vi "To XML - Returns XML Entities.vi"() -> ()   [LabVIEW 2017, in "Cobertura.Tests.lvlib" / "Class.lvlib"]
uses:
  Class.lvlib
  <vilib>/xml/Close Reference(Node).vi
  Cobertura/Class/Class.lvclass
  <vilib>/xml/NI_XML.lvlib
  <resource>/objmgr/DOMUserDefRef.rc
  <vilib>/PNR/Transparent Assertions/Transparent Assertions/Transparent Assertions.lvlib
panel:
  out "error out":errorcluster
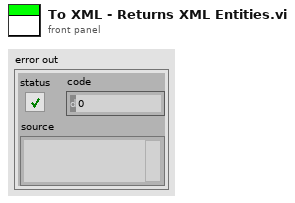
[diagram p1: front panel]
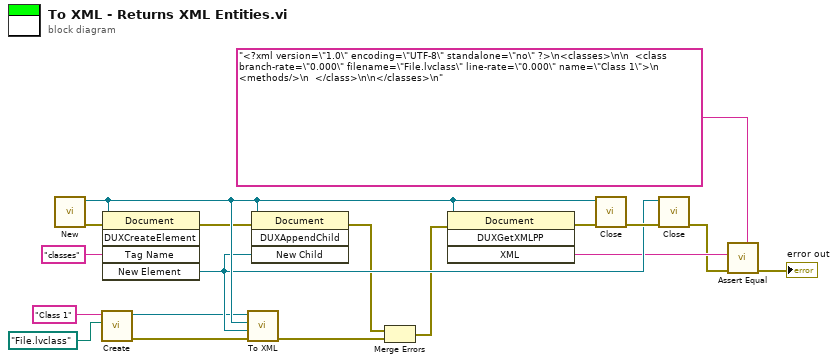
[diagram p0: block diagram]
diagram:
  n1 = call <vilib>:"New.vi"() -> ("error out"=w13:errorcluster, "DOM document out"=w15:refnum<k20>)  [unwired: 8 in]
  n2 = call "Create.vi"("Filename"=path "File.lvclass", "Name"="Class 1") -> ("error out"=w18:errorcluster, "Class"=w2:refnum<class "Class.lvclass">)  [unwired: 8 in]
  n3 = invoke class="Document" method="DUXCreateElement"(reference=w15, error in=w13, "Tag Name"="classes") -> (error out=w14:errorcluster, "New Element"=w11:refnum<k20>)  [unwired: 2 in, 3 out]
  n4 = call-dynamic "To XML.vi"("error in (no error)"=w18, "Parent"=w11, "Document"=w15, "Class in"=w2) -> ("error out"=w5:errorcluster)  [unwired: 7 in]
  n5 = invoke class="Document" method="DUXAppendChild"(reference=w15, error in=w14, "New Child"=w11) -> (error out=w7:errorcluster)  [unwired: 1 in, 3 out]
  n6 = Merge Errors(w7, w5) -> (w6:errorcluster)
  n7 = invoke class="Document" method="DUXGetXMLPP"(reference=w15, error in=w6) -> (error out=w16:errorcluster, "XML"=w10:string)  [unwired: 2 in, 2 out]
  n8 = call-poly <vilib>:"Close.vi"("error in (no error)"=w16, "node"=w15) -> ("error out"=w12:errorcluster)  [unwired: 7 in]
  n9 = call-poly <vilib>:"Close.vi"("error in (no error)"=w12, "node"=w11) -> ("error out"=w4:errorcluster)  [unwired: 7 in]
  n10 = call <vilib>:"Assert Equal.vi"("Expected"="<?xml version=\"1.0\" encoding=\"UTF-8\" standalone=\"no\" ?>\n<classes>\n\n  <class branch-rate=\"0.000\" filename=\"File.lvclass\" line-rate=\"0.000\" name=\"Class 1\">\n    <methods/>\n  </class>\n\n</classes>\n", "error in (no error)"=w4, "Actual"=w10) -> ("error out"=→"error out":errorcluster)  [unwired: 8 in]
